vi "BASE-Main.vi"() -> ()   [LabVIEW 2017]
uses:
  <vilib>/Utility/error.llb/DialogType.ctl
  55ed0eea-cd20-493f-8468-85b8c1a0a0c0.vi
  <vilib>/addons/database/Connection.llb/DB Tools Open Connec (Path).vi
  <vilib>/addons/database/NI_Database_API.lvlib
panel:
  in  "VARIENT 2":bool
  out "Status Number":i32
  out "Status":i32(ring)=1 items=["Stopped"=1, "StartPending"=2, "StopPending"=3, "Running"=4, "ContinuePending"=5, "PausePending"=6, "Paused"=7]
  in  "PRINT":bool
  out "error out":errorcluster
  in  "Logout":bool
  in  "Stop":bool
  in  "Create Login":bool
  in  "Reports":bool
  in  "Start":bool
  out "Time":string
  out "Date":string
  in  "Login":bool
  # "Py1b ORVM"
  # "UNIQUE CIRCLE\nAUTOMATION Pvt Ltd"
types:
  T1 = enum8{"Enabled", "Disabled", "Disabled and Grayed Out"}
  T2 = typedef "DialogType.ctl" = u16
  T3 = enum32{"Invalid", "Standard", "Closed", "Hidden", "Minimized", "Maximized"}
  T4 = typedef "NI_Database_API.lvlib/Conn ObjectReference.ctl" = refnum<k1>
  T5 = enum32{"invalid app kind", "Development System", "Run Time System", "Student Edition", "Embedded LabVIEW", "Evaluation", "Custom"}
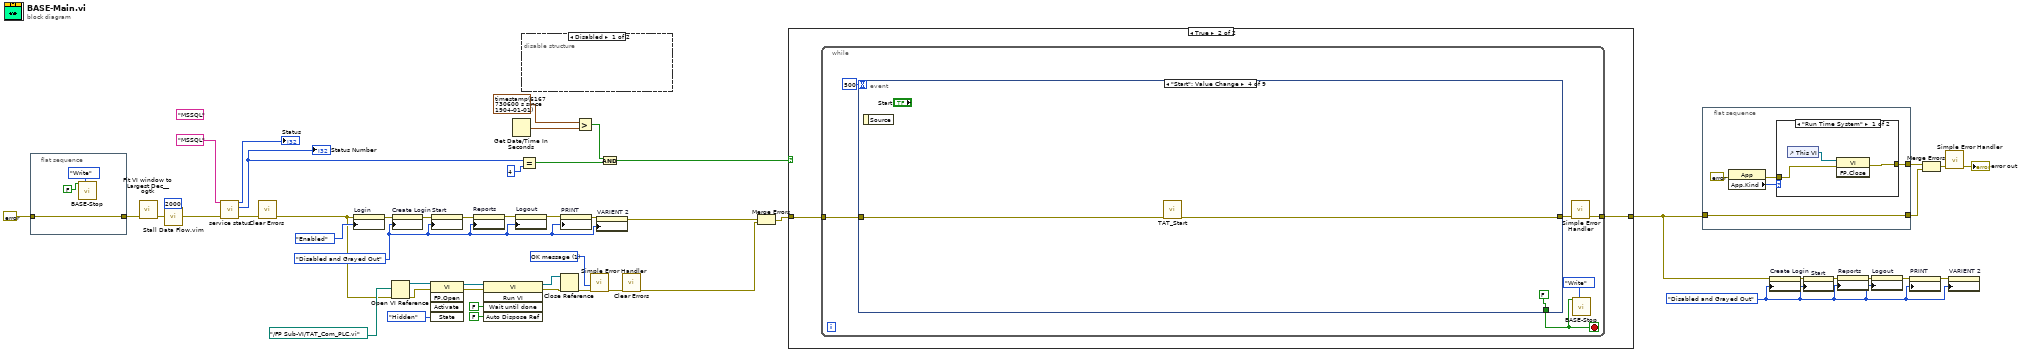
[diagram p0: block diagram]
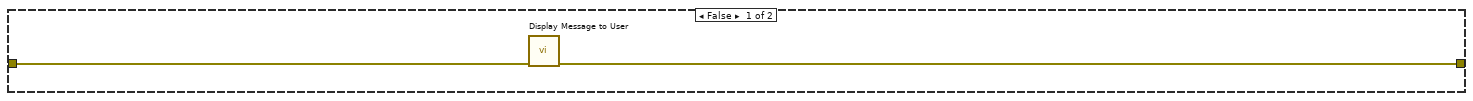
[diagram p4: hidden frame]
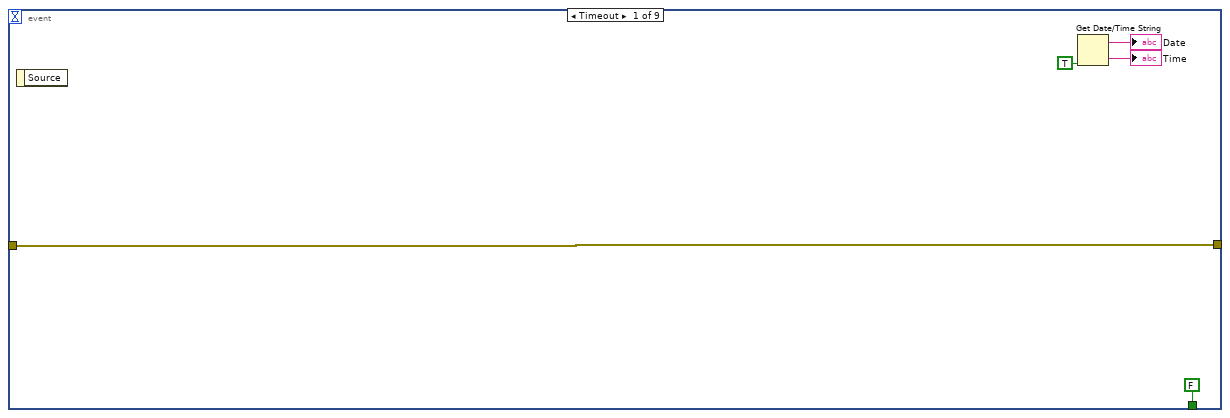
[diagram p5: hidden frame]
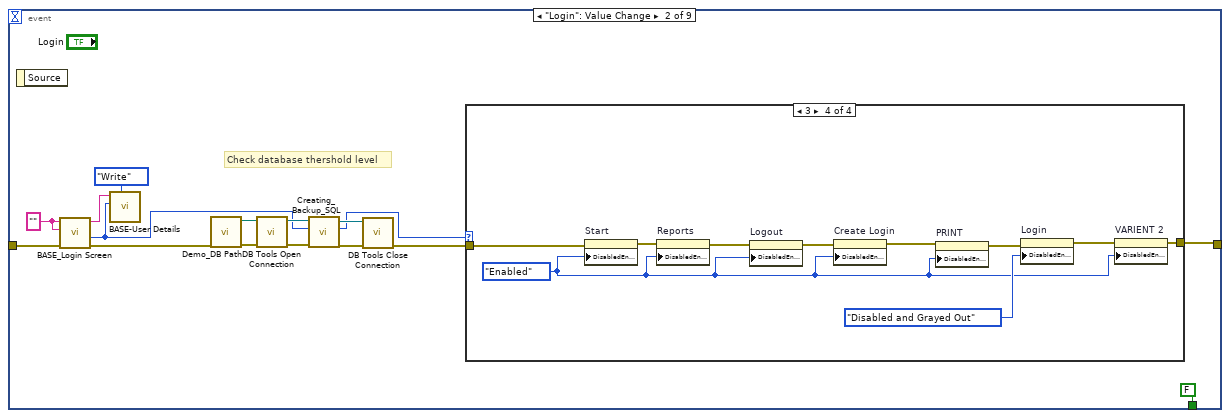
[diagram p6: hidden frame]
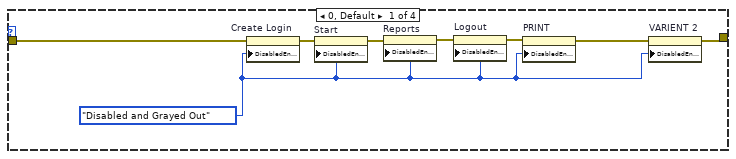
[diagram p7: hidden frame]
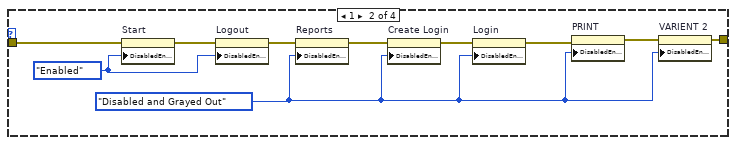
[diagram p8: hidden frame]
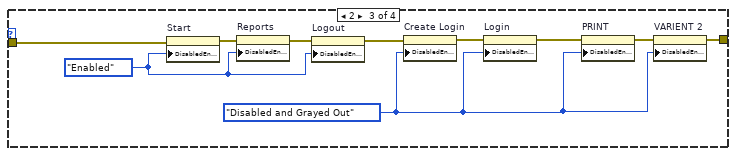
[diagram p9: hidden frame]
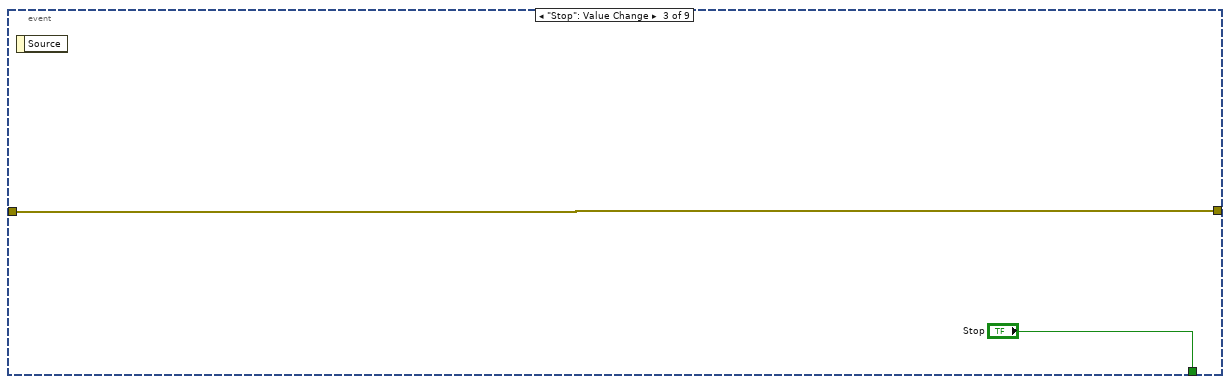
[diagram p10: hidden frame]
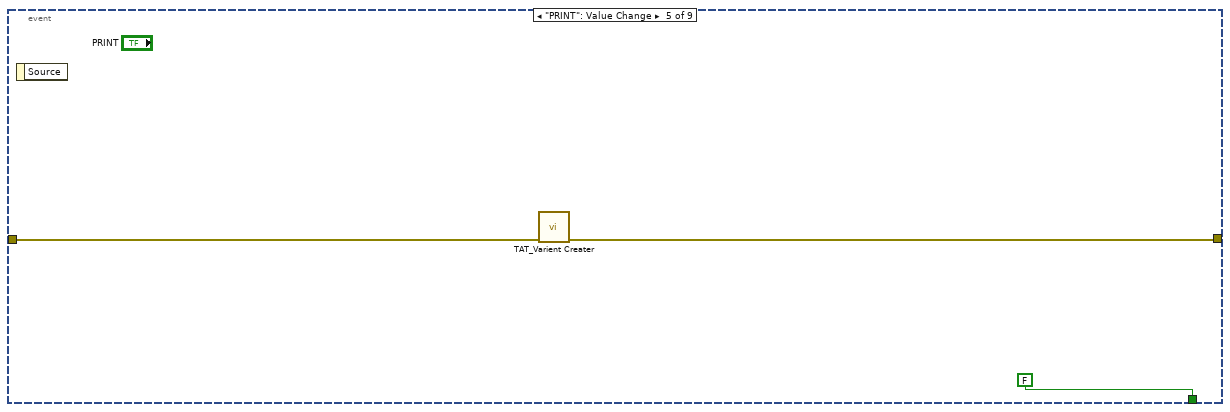
[diagram p11: hidden frame]
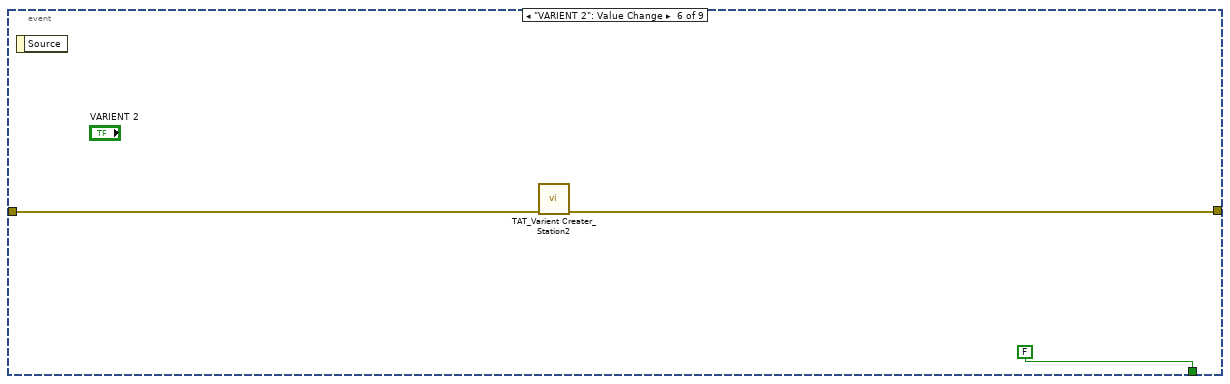
[diagram p12: hidden frame]
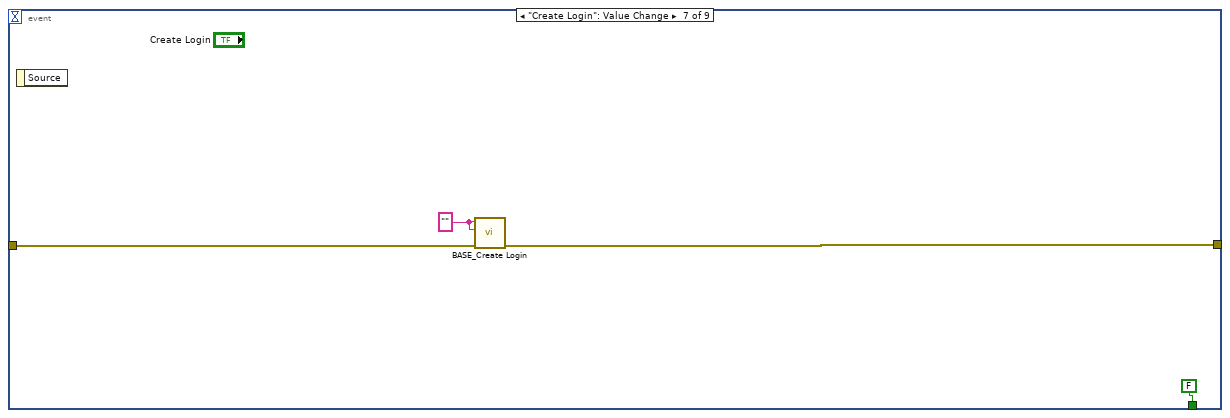
[diagram p13: hidden frame]
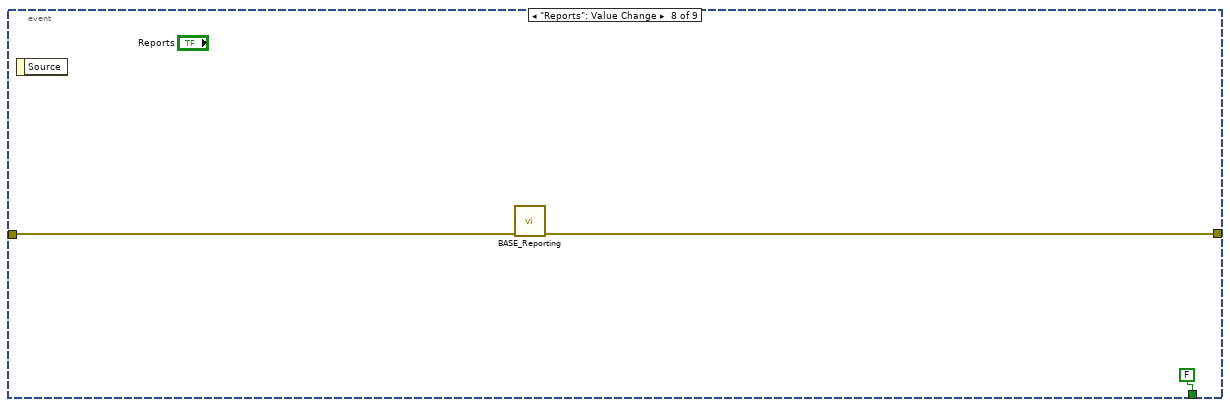
[diagram p14: hidden frame]
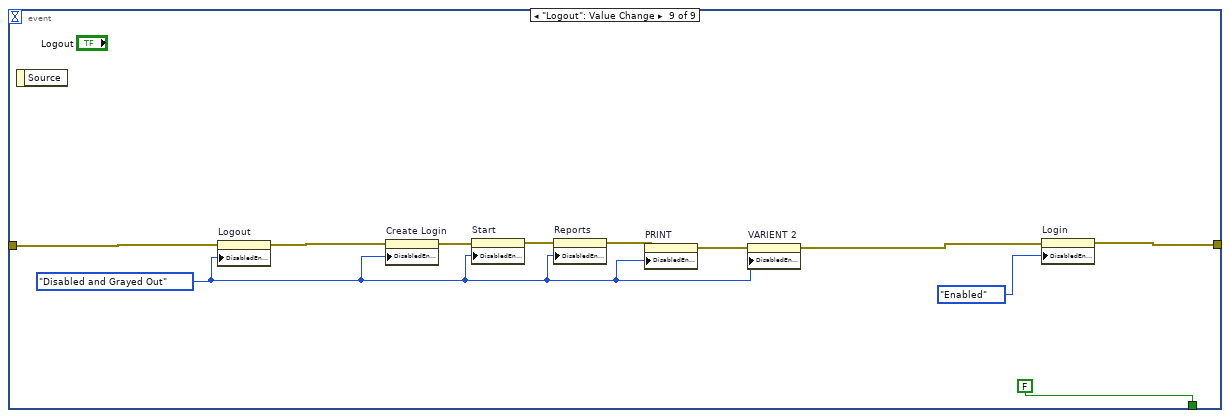
[diagram p15: hidden frame]
diagram:
  w2 = T1."Disabled and Grayed Out" ("Disabled")
  (unwired) "MSSQL" ("Service Name")
  w30 = T2 1 items=["no dialog", "OK message", "continue or stop message", "OK message + warnings", "continue/stop + warnings"] ("type of dialog (OK msg:1)")
  w3 = T1."Disabled and Grayed Out" ("Disabled")
  n1 = flat-sequence {
    tunnel: [w54] -> w43
    tunnel: errorcluster {"status"=FALSE, "code"=0, "source"=""} ("error constant") -> [w54]
    frame #0 {
      n2 = call "BASE-Stop.vi"("Enum"=enum16{"Read", "Write"}."Write", "Stop"=FALSE) -> ()  [unwired: 9 in, 1 out]
    }
  }
  n3 = call <userlib>:"Fit VI window to Largest Dec__ogtk.vi"("error in (no error)"=w43) -> ("error out"=w15:errorcluster)  [unwired: 5 in, 1 out]
  n4 = call "Stall Data Flow.vim"("value in"=w15, "milliseconds to wait"=u32 2000) -> ("value out"=w14:errorcluster)  [unwired: 1 out]
  n5 = call "service status.vi"("error in"=w14, "Service Name"="MSSQL") -> ("error out"=w22:errorcluster, "Status Number"=w24:i32, "Status"=→"Status":i32)  [unwired: 6 in, 1 out]
  "Status Number" <- w24
  n6 = call <vilib>:"Clear Errors.vi"("error in (no error)"=w22) -> ("error out"=w21:errorcluster)  [unwired: 5 in, 1 out]
  n7 = property on="Login" class="Bool"(error in=w21, "DisabledEnum"=T1."Enabled" ("Disabled")) -> (error out=w47:errorcluster)  [unwired: 1 in, 1 out]
  n8 = Open VI Reference(vi path=path "../FP Sub-VI/TAT_Com_PLC.vi", error in (no error)=w21) -> (vi reference=w39:refnum<vi>, error out=w40:errorcluster)  [unwired: 4 in]
  n9 = property on="Create Login" class="Bool"(error in=w47, "DisabledEnum"=w3) -> (error out=w51:errorcluster)  [unwired: 1 in, 1 out]
  n10 = invoke class="VI" method="FP.Open"(reference=w39, error in=w40, "State"=T3."Hidden") -> (reference out=w42:refnum<vi>, error out=w41:errorcluster)  [unwired: 2 in, 3 out]
  n11 = property on="Start" class="Bool"(error in=w51, "DisabledEnum"=w3) -> (error out=w11:errorcluster)  [unwired: 1 in, 1 out]
  n12 = property on="Reports" class="Bool"(error in=w11, "DisabledEnum"=w3) -> (error out=w45:errorcluster)  [unwired: 1 in, 1 out]
  n13 = invoke class="VI" method="Run VI"(reference=w42, error in=w41, "Wait until done"=FALSE ("Wait Until Done"), "Auto Dispose Ref"=FALSE ("Auto Dispose Reference")) -> (reference out=w38:refnum<vi>, error out=w37:errorcluster)  [unwired: 1 in, 3 out]
  n14 = Get Date/Time In Seconds() -> (seconds since 1Jan1904=w17:timestamp)
  n15 = property on="Logout" class="Bool"(error in=w45, "DisabledEnum"=w3) -> (error out=w12:errorcluster)  [unwired: 1 in, 1 out]
  n16 = Equal?(x=w24, y=4) -> (x = y?=w20:bool)
  n17 = disable-structure shown="Disabled" {
    frame Disabled {
    }
    frame Enabled {
    }
  }
  n18 = Close Reference(reference=w38, error in (no error)=w37) -> (error out=w31:errorcluster)
  n19 = property on="PRINT" class="Bool"(error in=w12, "DisabledEnum"=w3) -> (error out=w10:errorcluster)  [unwired: 1 in, 1 out]
  n20 = Greater?(x=timestamp(6167730600 s since 1904-01-01), y=w17) -> (0:w16:bool)
  n21 = call <vilib>:"Simple Error Handler.vi"("type of dialog (OK msg:1)"=w30, "error in (no error)"=w31) -> ("error out"=w29:errorcluster)  [unwired: 3 in, 4 out]
  n22 = property on="VARIENT 2" class="Bool"(error in=w10, "DisabledEnum"=w3) -> (error out=w1:errorcluster)  [unwired: 1 in, 1 out]
  n23 = And(x=w16, y=w20) -> (x .and. y?=w19:bool)
  n24 = call <vilib>:"Clear Errors.vi"("error in (no error)"=w29) -> ("error out"=w28:errorcluster)  [unwired: 5 in, 1 out]
  n25 = Merge Errors(w1, w28) -> (w33:errorcluster)
  n26 = case shown="True" w19 {
    tunnel: w33 -> [w56 w58]
    tunnel: [w55 w57] -> w4
    frame False {
      n27 = call "Display Message to User"("error in (no error)"=w56) -> ("error out"=w55:errorcluster)  [unwired: 9 in, 1 out]
    }
    frame True {
      n28 = while {
        tunnel: w58 -> [w63]
        tunnel: [w59] -> w57
        stop <- w60 stop-if-true
        n29 = event shown="[3] \"Start\": Value Change" {
          selector: _ -> [_ _ _ _ _ _ _ _ _]
          dyn-events: _ -> [_ _ _ _ _ _ _ _ _]
          timeout: 500 -> [_ _ _ _ _ _ _ _ _]
          tunnel: w63 -> [w67 w85 w124 w127 w130 w133 w138 w140 w149]
          tunnel: [w67 w80 w124 w126 w129 w132 w137 w139 w150] -> w62
          tunnel: [FALSE ("Stop") FALSE ("Stop") "Stop" FALSE ("Stop") FALSE ("Stop") FALSE ("Stop") FALSE ("Stop") FALSE ("Stop") FALSE ("Stop")] -> w60
          event Timeout {
            n30 = event-data() -> ()  [unwired: 1 in, 1 out]
            n31 = Get Date/Time String(want seconds? (F)=TRUE) -> (date string=→"Date":string, time string=→"Time":string)  [unwired: 2 in]
          }
          event "Login": Value Change {
            w82 = "" ("User Name")
            # "Check database thershold level"
            n32 = event-data() -> ()  [unwired: 1 in, 1 out]
            n33 = call "BASE_Login Screen.vi"("Error In"=w85, "Password"=w82, "User Name"=w82) -> ("error out"=w73:errorcluster, "Level"=w70:i32, "User Name Out"=w83:string)  [unwired: 5 in, 1 out]
            n34 = call "BASE-User Details.vi"("Enum"=enum16{"Read", "Write"}."Write", "Level In"=w70, "User Name In"=w83) -> ()  [unwired: 7 in, 2 out]
            n35 = call "Demo_DB Path.vi"("error in"=w73) -> ("error out"=w79:errorcluster, "DB Path"=w78:path)  [unwired: 9 in]
            n36 = call-poly <vilib>:"DB Tools Open Connection.vi"("error in (no error)"=w79, "connection information"=w78) -> ("error out"=w76:errorcluster, "connection reference"=w77:T4)  [unwired: 6 in]
            n37 = call "Creating_Backup_SQL.vi"("error in"=w76, "User level"=w70, "database in"=w77) -> ("error out"=w75:errorcluster, "User Level"=w71:i32, "Database out"=w74:T4)  [unwired: 6 in]
            n38 = call <vilib>:"DB Tools Close Connection.vi"("error in (no error)"=w75, "connection reference"=w74) -> ("error out"=w72:errorcluster)  [unwired: 5 in]
            n39 = case shown="3" w71 {
              tunnel: w72 -> [w91 w103 w113 w123]
              tunnel: [w86 w95 w104 w114] -> w80
              frame 0, Default {
                w87 = T1."Disabled and Grayed Out" ("Disabled")
                n40 = property on="Create Login" class="Bool"(error in=w91, "DisabledEnum"=w87) -> (error out=w93:errorcluster)  [unwired: 1 in, 1 out]
                n41 = property on="Start" class="Bool"(error in=w93, "DisabledEnum"=w87) -> (error out=w92:errorcluster)  [unwired: 1 in, 1 out]
                n42 = property on="Reports" class="Bool"(error in=w92, "DisabledEnum"=w87) -> (error out=w89:errorcluster)  [unwired: 1 in, 1 out]
                n43 = property on="Logout" class="Bool"(error in=w89, "DisabledEnum"=w87) -> (error out=w90:errorcluster)  [unwired: 1 in, 1 out]
                n44 = property on="PRINT" class="Bool"(error in=w90, "DisabledEnum"=w87) -> (error out=w88:errorcluster)  [unwired: 1 in, 1 out]
                n45 = property on="VARIENT 2" class="Bool"(error in=w88, "DisabledEnum"=w87) -> (error out=w86:errorcluster)  [unwired: 1 in, 1 out]
              }
              frame 1 {
                w94 = T1."Disabled and Grayed Out" ("Disabled")
                w96 = T1."Enabled" ("Disabled")
                n46 = property on="Start" class="Bool"(error in=w103, "DisabledEnum"=w96) -> (error out=w99:errorcluster)  [unwired: 1 in, 1 out]
                n47 = property on="Logout" class="Bool"(error in=w99, "DisabledEnum"=w96) -> (error out=w101:errorcluster)  [unwired: 1 in, 1 out]
                n48 = property on="Reports" class="Bool"(error in=w101, "DisabledEnum"=w94) -> (error out=w102:errorcluster)  [unwired: 1 in, 1 out]
                n49 = property on="Create Login" class="Bool"(error in=w102, "DisabledEnum"=w94) -> (error out=w100:errorcluster)  [unwired: 1 in, 1 out]
                n50 = property on="Login" class="Bool"(error in=w100, "DisabledEnum"=w94) -> (error out=w98:errorcluster)  [unwired: 1 in, 1 out]
                n51 = property on="PRINT" class="Bool"(error in=w98, "DisabledEnum"=w94) -> (error out=w97:errorcluster)  [unwired: 1 in, 1 out]
                n52 = property on="VARIENT 2" class="Bool"(error in=w97, "DisabledEnum"=w94) -> (error out=w95:errorcluster)  [unwired: 1 in, 1 out]
              }
              frame 2 {
                w105 = T1."Disabled and Grayed Out" ("Disabled")
                w106 = T1."Enabled" ("Disabled")
                n53 = property on="Start" class="Bool"(error in=w113, "DisabledEnum"=w106) -> (error out=w110:errorcluster)  [unwired: 1 in, 1 out]
                n54 = property on="Reports" class="Bool"(error in=w110, "DisabledEnum"=w106) -> (error out=w112:errorcluster)  [unwired: 1 in, 1 out]
                n55 = property on="Logout" class="Bool"(error in=w112, "DisabledEnum"=w106) -> (error out=w108:errorcluster)  [unwired: 1 in, 1 out]
                n56 = property on="Create Login" class="Bool"(error in=w108, "DisabledEnum"=w105) -> (error out=w111:errorcluster)  [unwired: 1 in, 1 out]
                n57 = property on="Login" class="Bool"(error in=w111, "DisabledEnum"=w105) -> (error out=w109:errorcluster)  [unwired: 1 in, 1 out]
                n58 = property on="PRINT" class="Bool"(error in=w109, "DisabledEnum"=w105) -> (error out=w107:errorcluster)  [unwired: 1 in, 1 out]
                n59 = property on="VARIENT 2" class="Bool"(error in=w107, "DisabledEnum"=w105) -> (error out=w104:errorcluster)  [unwired: 1 in, 1 out]
              }
              frame 3 {
                w115 = T1."Enabled" ("Disabled")
                n60 = property on="Start" class="Bool"(error in=w123, "DisabledEnum"=w115) -> (error out=w118:errorcluster)  [unwired: 1 in, 1 out]
                n61 = property on="Reports" class="Bool"(error in=w118, "DisabledEnum"=w115) -> (error out=w122:errorcluster)  [unwired: 1 in, 1 out]
                n62 = property on="Logout" class="Bool"(error in=w122, "DisabledEnum"=w115) -> (error out=w121:errorcluster)  [unwired: 1 in, 1 out]
                n63 = property on="Create Login" class="Bool"(error in=w121, "DisabledEnum"=w115) -> (error out=w120:errorcluster)  [unwired: 1 in, 1 out]
                n64 = property on="PRINT" class="Bool"(error in=w120, "DisabledEnum"=w115) -> (error out=w119:errorcluster)  [unwired: 1 in, 1 out]
                n65 = property on="Login" class="Bool"(error in=w119, "DisabledEnum"=T1."Disabled and Grayed Out" ("Disabled")) -> (error out=w117:errorcluster)  [unwired: 1 in, 1 out]
                n66 = property on="VARIENT 2" class="Bool"(error in=w117, "DisabledEnum"=w115) -> (error out=w114:errorcluster)  [unwired: 1 in, 1 out]
              }
            }
          }
          event "Stop": Value Change {
            n67 = event-data() -> ()  [unwired: 1 in, 1 out]
          }
          event "Start": Value Change {
            n68 = event-data() -> ()  [unwired: 1 in, 1 out]
            n69 = call "TAT_Start.vi"("error In"=w127) -> ("error out"=w126:errorcluster)  [unwired: 10 in]
          }
          event "PRINT": Value Change {
            n70 = event-data() -> ()  [unwired: 1 in, 1 out]
            n71 = call "TAT_Varient Creater.vi"("error in (no error)"=w130) -> ("error out"=w129:errorcluster)  [unwired: 10 in]
          }
          event "VARIENT 2": Value Change {
            n72 = event-data() -> ()  [unwired: 1 in, 1 out]
            n73 = call "TAT_Varient Creater_Station2.vi"("error in (no error)"=w133) -> ("error out"=w132:errorcluster)  [unwired: 10 in]
          }
          event "Create Login": Value Change {
            w136 = "" ("User Name")
            n74 = event-data() -> ()  [unwired: 1 in, 1 out]
            n75 = call "BASE_Create Login.vi"("Error In"=w138, "Password"=w136, "User Name"=w136) -> ("error out"=w137:errorcluster)  [unwired: 6 in]
          }
          event "Reports": Value Change {
            n76 = event-data() -> ()  [unwired: 1 in, 1 out]
            n77 = call "BASE_Reporting.vi"("error in (no error)"=w140) -> ("error out"=w139:errorcluster)  [unwired: 10 in]
          }
          event "Logout": Value Change {
            w144 = T1."Disabled and Grayed Out" ("Disabled")
            n78 = event-data() -> ()  [unwired: 1 in, 1 out]
            n79 = property on="Logout" class="Bool"(error in=w149, "DisabledEnum"=w144) -> (error out=w145:errorcluster)  [unwired: 1 in, 1 out]
            n80 = property on="Create Login" class="Bool"(error in=w145, "DisabledEnum"=w144) -> (error out=w152:errorcluster)  [unwired: 1 in, 1 out]
            n81 = property on="Start" class="Bool"(error in=w152, "DisabledEnum"=w144) -> (error out=w151:errorcluster)  [unwired: 1 in, 1 out]
            n82 = property on="Reports" class="Bool"(error in=w151, "DisabledEnum"=w144) -> (error out=w146:errorcluster)  [unwired: 1 in, 1 out]
            n83 = property on="PRINT" class="Bool"(error in=w146, "DisabledEnum"=w144) -> (error out=w143:errorcluster)  [unwired: 1 in, 1 out]
            n84 = property on="VARIENT 2" class="Bool"(error in=w143, "DisabledEnum"=w144) -> (error out=w142:errorcluster)  [unwired: 1 in, 1 out]
            n85 = property on="Login" class="Bool"(error in=w142, "DisabledEnum"=T1."Enabled" ("Disabled")) -> (error out=w150:errorcluster)  [unwired: 1 in, 1 out]
          }
        }
        n86 = call <vilib>:"Simple Error Handler.vi"("error in (no error)"=w62) -> ("error out"=w59:errorcluster)  [unwired: 4 in, 4 out]
        n87 = call "BASE-Stop.vi"("Enum"=enum16{"Read", "Write"}."Write", "Stop"=w60) -> ()  [unwired: 9 in, 1 out]
      }
    }
  }
  n88 = flat-sequence {
    tunnel: [w154] -> w50
    tunnel: [w153] -> w48
    tunnel: w4 -> [w153]
    frame #0 {
      n89 = property class="App"(error in=errorcluster {"status"=FALSE, "code"=0, "source"=""} ("error in (no error)")) -> (error out=w156:errorcluster, "App.Kind"=w157:T5)  [unwired: 1 in, 1 out]
      n90 = case shown="\"Run Time System\"" w157 {
        tunnel: w156 -> [w159 w161]
        tunnel: [w158 w161] -> w154
        frame "Run Time System" {
          n91 = control-ref of="This VI"() -> (w160:refnum<vi>)
          n92 = invoke class="VI" method="FP.Close"(reference=w160, error in=w159) -> (error out=w158:errorcluster)  [unwired: 1 in, 2 out]
        }
        frame "Development System", Default {
        }
      }
    }
  }
  n93 = property on="Create Login" class="Bool"(error in=w4, "DisabledEnum"=w2) -> (error out=w5:errorcluster)  [unwired: 1 in, 1 out]
  n94 = property on="Start" class="Bool"(error in=w5, "DisabledEnum"=w2) -> (error out=w8:errorcluster)  [unwired: 1 in, 1 out]
  n95 = property on="Reports" class="Bool"(error in=w8, "DisabledEnum"=w2) -> (error out=w6:errorcluster)  [unwired: 1 in, 1 out]
  n96 = property on="Logout" class="Bool"(error in=w6, "DisabledEnum"=w2) -> (error out=w7:errorcluster)  [unwired: 1 in, 1 out]
  n97 = property on="PRINT" class="Bool"(error in=w7, "DisabledEnum"=w2) -> (error out=w9:errorcluster)  [unwired: 1 in, 1 out]
  n98 = Merge Errors(w50, w48) -> (w49:errorcluster)
  n99 = call <vilib>:"Simple Error Handler.vi"("error in (no error)"=w49) -> ("error out"=→"error out":errorcluster)  [unwired: 4 in, 4 out]
  n100 = property on="VARIENT 2" class="Bool"(error in=w9, "DisabledEnum"=w2) -> ()  [unwired: 1 in, 2 out]
